vi "Cascade.vi"(8 "Error In":errorcluster, 9 "Vertical Step":i16=20 caption="Vertical Step (20)", 10 "Horizontal Step":i16=20 caption="Horizontal Step (20)", 11 "Cascade":string="Default" caption="Cascade Group ('Default')") -> (0 "Error Out":errorcluster, 3 "Cascade out":refnum<class "Cascade.lvclass">)   [LabVIEW 2019, in "Panel.lvlib" / "Cascade.lvclass"]
doc: "Automatically cascades the windows.\n\nWindows in the same Cascade Group won't be placed on top of each other.\n\n<B>Cascade Group:</B> Specifies the cascade group\n<B>Horizontal Step:</B> Defines the horizontal cascade step.\n<B>Vertical Step:</B> Defines the vertical cascade step.\n<B>Error In:</B> Describes error conditions that occur before this node runs.\n\n<B>Cascade Out:</B> Cascade object.\n<B>Error Out:</B> Contains error information.\n\n----\nPlease see the following web address for additional documentation and tutorial information:\nhttp://www.mooregoodideas.com/mgi-panel-manager/\n\nAuthor: Derek Trepanier\n\nCopyright (c) 2018, Moore Good Ideas, Inc.\n\nAll rights reserved.\n\nRedistribution and use in source and binary forms, with or without modification, are permitted provided that the following conditions are met:\n\n * Redistributions of source code must retain the above copyright notice, this list of conditions and the following disclaimer.\n * Redistributions in binary form must reproduce the above copyright notice, this list of conditions and the following disclaimer in the documentation and/or other materials provided with the distribution.\n * Neither the name of Moore Good Ideas, Inc. nor the names of its contributors may be used to endorse or promote products derived from this software without specific prior written permission.\n\nTHIS SOFTWARE IS PROVIDED BY THE COPYRIGHT HOLDERS AND CONTRIBUTORS \"AS IS\" AND ANY EXPRESS OR IMPLIED WARRANTIES, INCLUDING, BUT NOT LIMITED TO, THE IMPLIED WARRANTIES OF MERCHANTABILITY AND FITNESS FOR A PARTICULAR PURPOSE ARE DISCLAIMED. IN NO EVENT SHALL THE COPYRIGHT OWNER OR CONTRIBUTORS BE LIABLE FOR ANY DIRECT, INDIRECT, INCIDENTAL, SPECIAL, EXEMPLARY, OR CONSEQUENTIAL DAMAGES (INCLUDING, BUT NOT LIMITED TO, PROCUREMENT OF SUBSTITUTE GOODS OR SERVICES; LOSS OF USE, DATA, OR PROFITS; OR BUSINESS INTERRUPTION) HOWEVER CAUSED AND ON ANY THEORY OF LIABILITY, WHETHER IN CONTRACT, STRICT LIABILITY, OR TORT (INCLUDING NEGLIGENCE OR OTHERWISE) ARISING IN ANY WAY OUT OF THE USE OF THIS SOFTWARE, EVEN IF ADVISED OF THE POSSIBILITY OF SUCH DAMAGE."
uses:
  Cascade.lvclass
  Cascade.lvclass/Cascade.ctl
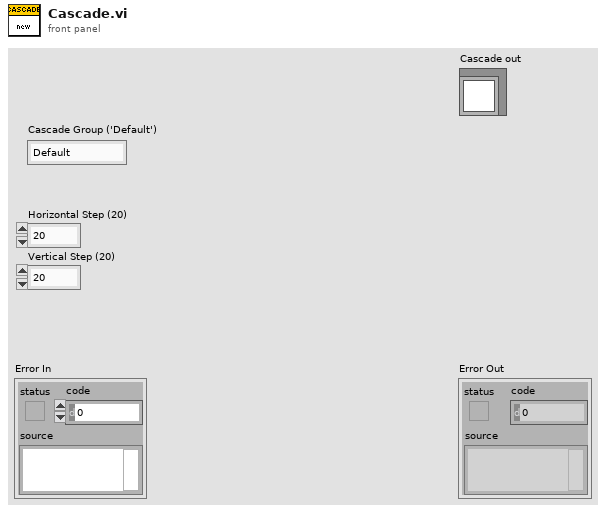
[diagram p1: front panel]
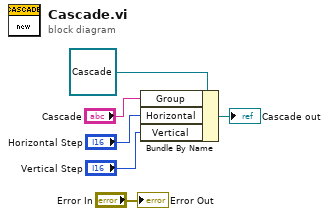
[diagram p0: block diagram]
diagram:
  n1 = Bundle By Name(cluster=refnum<class "Cascade.lvclass"> refnum ("Cascade in"), "Group"="Cascade", "Horizontal"="Horizontal Step", "Vertical"="Vertical Step") -> (→"Cascade out":refnum<class "Cascade.lvclass">)
  "Error Out" <- "Error In"
